vi "Tank.vi"() -> (2 "right velocity":dbl[](array[numeric]), 3 "left velocity":dbl[](array[numeric]))   [LabVIEW 2018]
uses:
  Pathfinder-Lib/VIs/Waypoint.ctl
  Pathfinder-Lib/Pathfinder.lvlib
panel:
  in  "Tab Control":enum32{"Primary Path", "Tank Position"}(tab)=enum."Tank Position"
  out "Path":T1(graph)
  out "Position":cluster{dbl[], dbl[]}[](graph)
  out "error out":errorcluster
  in  "wheelbase_width":dbl=24.0
  in  "sample_count":i32=1000
  in  "dt":dbl=0.001
  in  "max_jerk":dbl=60.0
  in  "max_acceleration":dbl=10.0
  in  "max_velocity":dbl=15.0
  in  "path":T2[](array[typedef])=[{"x"=12.0, "y"=60.0, "angle"=0.0}, {"x"=132.0, "y"=125.0, "angle"=60.0}]
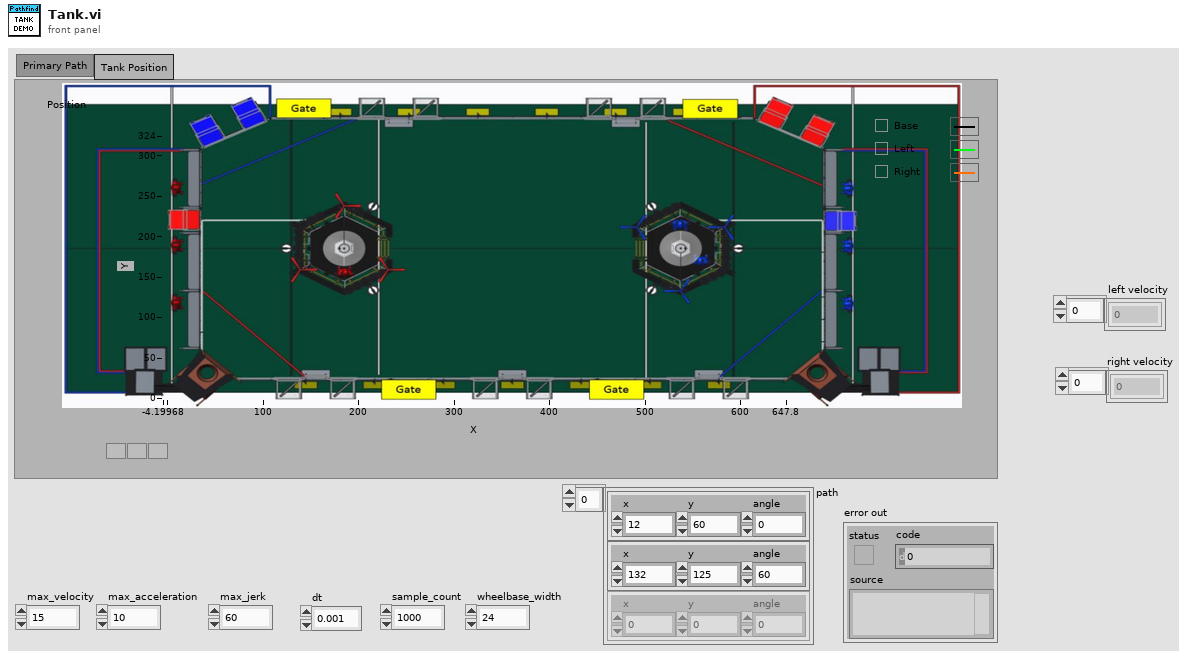
[diagram p1: front panel]
types:
  T1 = cluster{"position":dbl, "velocity":dbl, "acceleration":dbl, "jerk":dbl, "heading":dbl}[]
  T2 = typedef "Pathfinder.lvlib/Waypoint.ctl" = cluster{"x":dbl, "y":dbl, "angle":dbl}
  T3 = typedef "Pathfinder.lvlib/Segment.ctl" = cluster{"dt":dbl, "x":dbl, "y":dbl, "position":dbl, "velocity":dbl, "acceleration":dbl, "jerk":dbl, "heading":dbl}
  T4 = cluster{"position":dbl, "velocity":dbl, "acceleration":dbl, "jerk":dbl, "heading":dbl}
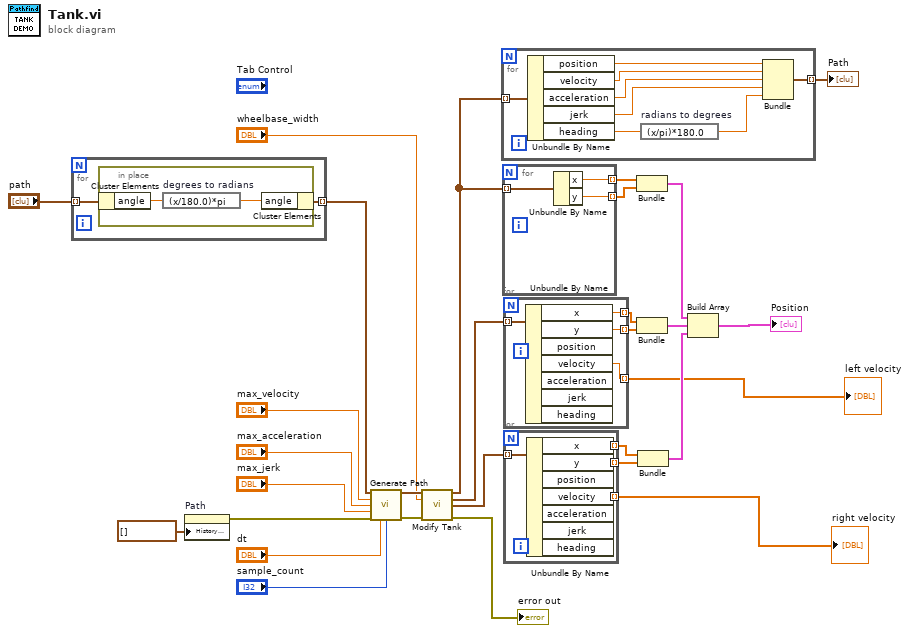
[diagram p0: block diagram]
diagram:
  n1 = for {
    tunnel: "path" -> [w31] mode=indexing
    tunnel: [w30] -> w4 mode=indexing
    n2 = in-place {
      n3 = in-place-cluster #1(w31) -> ("angle"=w33:dbl)
      n4 = expression code="(x/180.0)*pi" "degrees to radians"(w33) -> (w32:dbl)
      n5 = in-place-cluster #1("angle"=w32) -> (w30:T2)
    }
  }
  n6 = property on="Path" class="WFChart (strict)"("History Data"=T1 []) -> (error out=w6:errorcluster)  [unwired: 2 in, 1 out]
  n7 = call "Generate Path.vi"("path"=w4, "max_velocity"="max_velocity", "max_acceleration"="max_acceleration", "max_jerk"="max_jerk", "error in"=w6, "dt (.001)"="dt", "sample_count (100000)"="sample_count") -> ("Segments"=w29:T3[], "error out"=w25:errorcluster)  [unwired: 7 in]
  n8 = call "Modify Tank.vi"("Original"=w29, "wheelbase_width"="wheelbase_width", "error in"=w25) -> ("original"=w11:T3[], "left"=w20:T3[], "right"=w19:T3[], "error out"=→"error out":errorcluster)  [unwired: 9 in]
  n9 = for {
    tunnel: w11 -> [w41] mode=indexing
    tunnel: [w35] -> w21 mode=indexing
    n10 = Unbundle By Name(w41) -> ("position"=w40:dbl, "velocity"=w39:dbl, "acceleration"=w38:dbl, "jerk"=w37:dbl, "heading"=w36:dbl)
    n11 = expression code="(x/pi)*180.0" "radians to degrees"(w36) -> (w34:dbl)
    n12 = Bundle("position"=w40, "velocity"=w39, "acceleration"=w38, "jerk"=w37, "heading"=w34) -> (w35:T4)  [unwired: 1 in]
  }
  "Path" <- w21
  n13 = for {
    tunnel: w11 -> [w44] mode=indexing
    tunnel: [w43] -> w10 mode=indexing
    tunnel: [w42] -> w9 mode=indexing
    n14 = Unbundle By Name(w44) -> ("x"=w43:dbl, "y"=w42:dbl)
  }
  n15 = for {
    tunnel: w20 -> [w48] mode=indexing
    tunnel: [w47] -> w18 mode=indexing
    tunnel: [w46] -> w17 mode=indexing
    tunnel: [w45] -> w2 mode=indexing
    n16 = Unbundle By Name(w48) -> ("x"=w47:dbl, "y"=w46:dbl, "velocity"=w45:dbl)  [unwired: 4 out]
  }
  "left velocity" <- w2
  n17 = for {
    tunnel: w19 -> [w52] mode=indexing
    tunnel: [w51] -> w16 mode=indexing
    tunnel: [w50] -> w15 mode=indexing
    tunnel: [w49] -> w1 mode=indexing
    n18 = Unbundle By Name(w52) -> ("x"=w51:dbl, "y"=w50:dbl, "velocity"=w49:dbl)  [unwired: 4 out]
  }
  "right velocity" <- w1
  n19 = Bundle(w10, w9) -> (w8:cluster{dbl[], dbl[]})  [unwired: 1 in]
  n20 = Bundle(w18, w17) -> (w13:cluster{dbl[], dbl[]})  [unwired: 1 in]
  n21 = Bundle(w16, w15) -> (w14:cluster{dbl[], dbl[]})  [unwired: 1 in]
  n22 = Build Array(w8, w13, w14) -> (→"Position":cluster{dbl[], dbl[]}[])
